vi "sub_数组大小取最小值整数倍.vi"(3 "Input":i16[](array[numeric])) -> (1 "Output":i16[](array[numeric]), 2 "最小值":i16)   [LabVIEW 2015]
uses:
  <userlib>/_OpenG.lib/array/array.llb/Search 1D Array (I16)__ogtk.vi
panel:
  out "Indices of Elements":i32[](array[numeric])
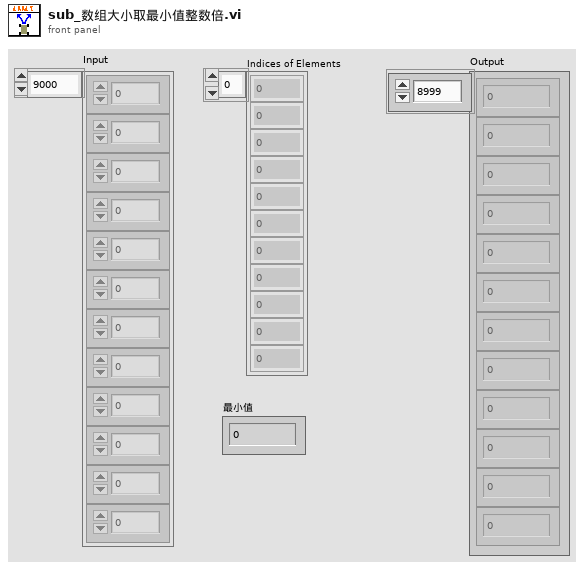
[diagram p1: front panel]
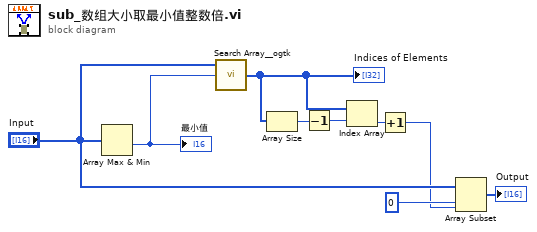
[diagram p0: block diagram]
diagram:
  n1 = Array Max & Min(array="Input") -> (min value=w7:i16)  [unwired: 3 out]
  "最小值" <- w7
  n2 = call-poly <userlib>:"Search Array__ogtk.vi"("Array"="Input", "Element Data"=w7) -> ("Indices of Elements"=w5:i32[])  [unwired: 7 in]
  "Indices of Elements" <- w5
  n3 = Array Size(array=w5) -> (size(s)=w6:i32)
  n4 = Decrement(x=w6) -> (x-1=w4:i32)
  n5 = Index Array(array=w5, index=w4) -> (element=w3:i32)
  n6 = Increment(x=w3) -> (x+1=w1:i32)
  n7 = Array Subset(array="Input", index=0 ("索引"), length=w1) -> (→"Output":i16[])
